vi "ReadSilos.vi"(9 "AIN Channel":dbl, 10 "Remote Port":u16=502, 11 "Remote IP Address":string="192.168.126.147") -> (0 "READ_D : PERIOD":sgl, 1 "READ_C : AVERAGE":sgl=0.912965, 2 "READ_B : RANGE":sgl=3.2546682, 3 "READ_A : RMS":sgl=1.7184298)   [LabVIEW 2022 SP3]
doc: "The LabJack T7 offers several AIN Extended Features. One such feature is called FlexRMS. Data acquired at a specified AIN Channel are buffered, on-board calculations (rms,range,average) are performed and the results are written to AIN-EF registers. This VI makes use of the EF to avoid using external computational resources whilst seeking averaged data. One noteworthy caveat is that the register containing the averaged data does not update unless the rms register is read."
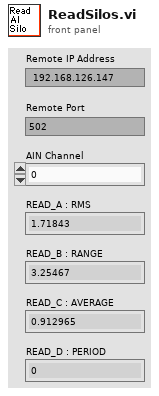
[diagram p1: front panel]
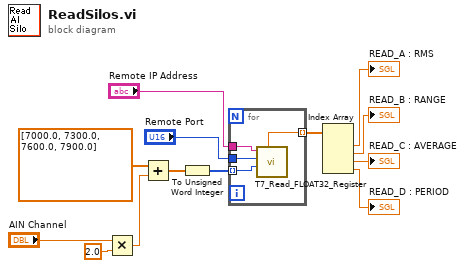
[diagram p0: block diagram]
diagram:
  n1 = Multiply(x="AIN Channel", y=2.0) -> (x*y=w3:dbl)
  n2 = Add(x=dbl[] [7000.0, 7300.0, 7600.0, 7900.0], y=w3) -> (x+y=w10:dbl[])
  n3 = To Unsigned Word Integer(number=w10) -> (unsigned 16bit integer=w9:u16[])
  n4 = for {
    tunnel: w9 -> [w17] mode=indexing
    tunnel: [w16] -> w8 mode=indexing
    tunnel: "Remote Port" -> [w15]
    tunnel: "Remote IP Address" -> [w14]
    n5 = call "T7_Read_FLOAT32_Register.vi"("LabJack TestFLOAT32 Register"=w17, "Remote Port"=w15, "Remote IP Address"=w14) -> ("Read FLOAT32"=w16:sgl)  [unwired: 7 in, 1 out]
  }
  n6 = Index Array(array=w8) -> (element #1=→"READ_A : RMS":sgl, element #2=→"READ_B : RANGE":sgl, element #3=→"READ_C : AVERAGE":sgl, element #4=→"READ_D : PERIOD":sgl)  [unwired: 4 in]
